vi "LWXPS_ControllerStatusStringGet.vi"(0 "XPS Reference IN":refnum<k24>, 7 "Controller Status Code":i32, 11 "LabVIEW error IN":errorcluster) -> (4 "XPS Reference OUT":refnum<k24>, 6 "Returned error code":i32, 8 "Controller Status String":string, 10 "XPS Error String":string, 15 "LabVIEW error OUT":errorcluster)   [LabVIEW 2014]
uses:
  D:/XPSQ8_LabView_Library/Development/Source/Dll/Newport.XPS.CommandInterface.dll
  Dll/Newport.XPS.CommandInterface.dll
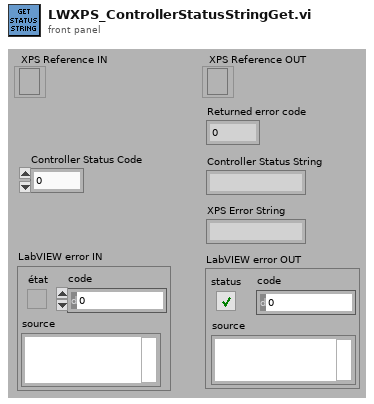
[diagram p1: front panel]
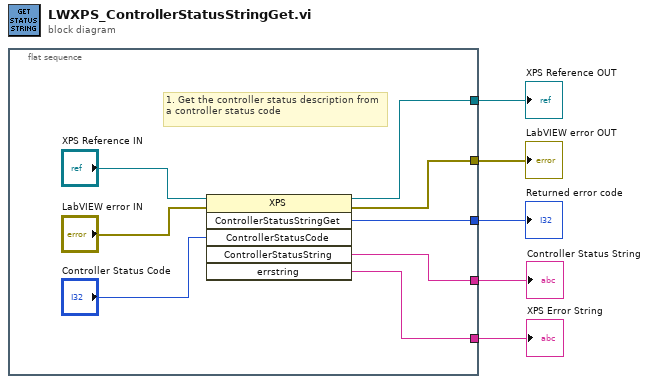
[diagram p0: block diagram]
diagram:
  n1 = flat-sequence {
    tunnel: [w9] -> w5
    tunnel: [w13] -> w4
    tunnel: [w10] -> w3
    tunnel: [w8] -> w2
    tunnel: [w6] -> w1
    frame #0 {
      # "1. Get the controller status description from a controller status code"
      n2 = invoke class="XPS" method="ControllerStatusStringGet"(reference="XPS Reference IN", error in="LabVIEW error IN", "ControllerStatusCode"="Controller Status Code") -> (reference out=w9:refnum<k24>, error out=w13:errorcluster, "ControllerStatusStringGet"=w10:i32, "ControllerStatusString"=w8:string, "errstring"=w6:string)  [unwired: 3 in, 1 out]
    }
  }
  "XPS Reference OUT" <- w5
  "LabVIEW error OUT" <- w4
  "Returned error code" <- w3
  "Controller Status String" <- w2
  "XPS Error String" <- w1
